vi "Get Class Types to Parent--recursive.vi"(6 "Application Ref":refnum<vi>, 7 "Class Level To Reach":refnum<class>, 8 "error in (no error)":errorcluster, 11 "Instance":refnum<class>) -> (0 "error out":errorcluster, 2 "Class Levels To Requested (FQN)":string[](array[string]), 3 "Class Levels To Requested (Types)":refnum<class>[](array[class]))   [LabVIEW 2019, in "Class Integrator.lvlib"]
uses:
  Class Integrator.lvlib
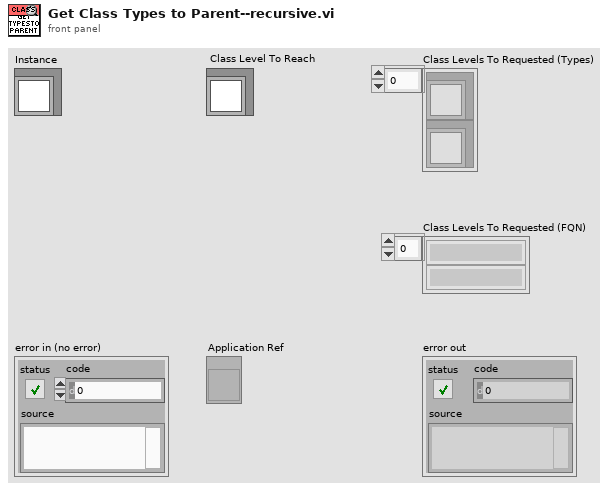
[diagram p1: front panel]
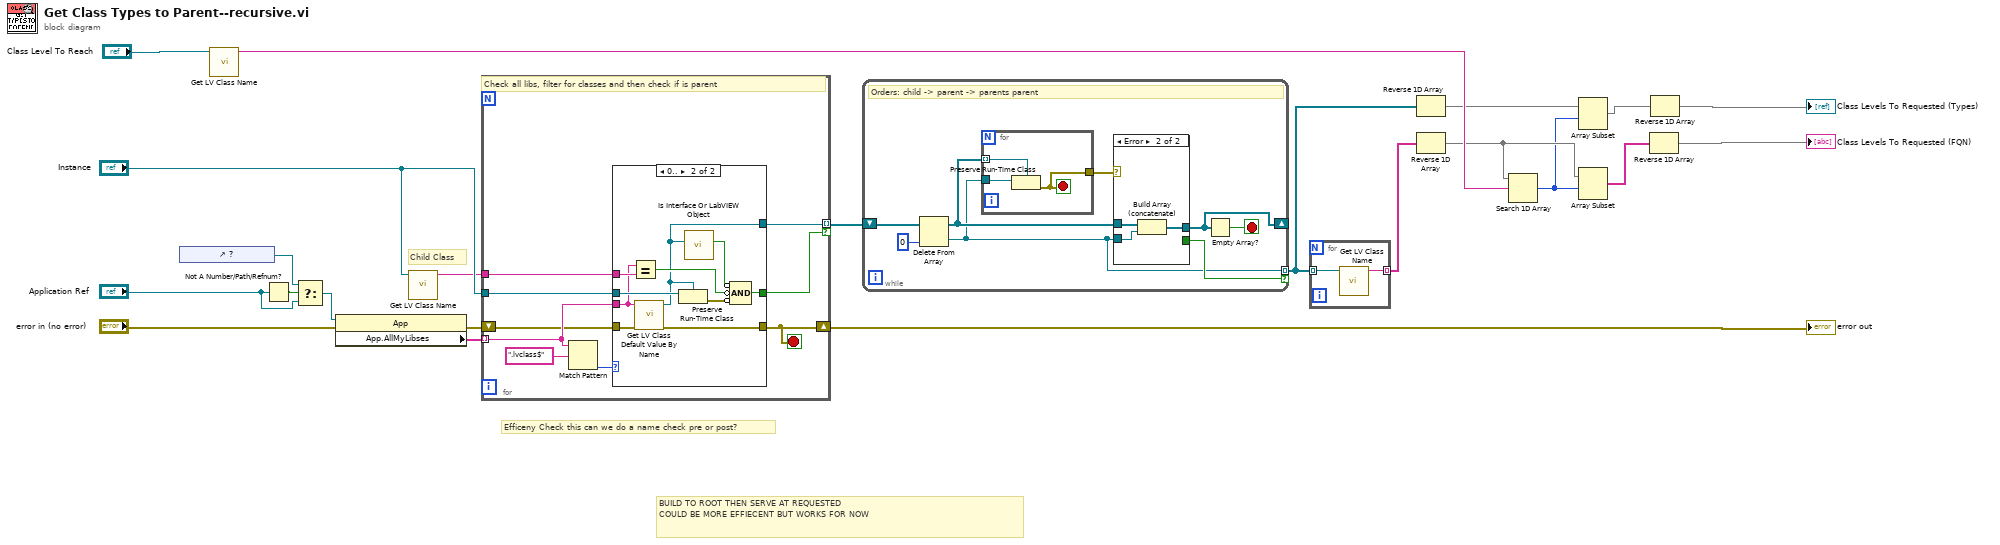
[diagram p0: block diagram]
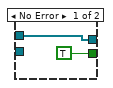
[diagram p3: hidden frame]
diagram:
  # "BUILD TO ROOT THEN SERVE AT REQUESTED\nCOULD BE MORE EFFIECENT BUT WORKS FOR NOW"
  # "Efficeny Check this can we do a name check pre or post?"
  # "Child Class"
  n1 = control-ref of="?"() -> (w14:refnum<vi>)
  n2 = call <vilib>:"Get LV Class Name.vi"("object"="Class Level To Reach") -> ("class name"=w8:string)  [unwired: 9 in, 1 out]
  n3 = Not A Number/Path/Refnum?(number/path/refnum="Application Ref") -> (NaN/Path/Refnum?=w15:bool)
  n4 = Select(t=w14, s=w15, f="Application Ref") -> (s? t:f=w9:refnum<vi>)
  n5 = property class="App"(reference=w9, error in="error in (no error)") -> (error out=w11:errorcluster, "App.AllMyLibses"=w10:string[])  [unwired: 1 out]
  n6 = call <vilib>:"Get LV Class Name.vi"("object"="Instance") -> ("class name"=w12:string)  [unwired: 9 in, 1 out]
  n7 = for {
    tunnel: w10 -> [w31] mode=indexing
    tunnel: [w26] -> w13 mode=indexing if=w25
    shift-right: [w27] -> w22
    shift-left: w11 -> [w28]
    tunnel: "Instance" -> [w24]
    tunnel: w12 -> [w23]
    stop <- w27 stop-if-true
    # "Check all libs, filter for classes and then check if is parent"
    n8 = Match Pattern(string=w31, regular expression=".lvclass$") -> (offset past match=w30:i32)  [unwired: 1 in, 3 out]
    n9 = case shown="0.." w30 {
      tunnel: [_ w33] -> w26
      tunnel: w31 -> [_ w36]
      tunnel: [_ w41] -> w25
      tunnel: [_ w40] -> w27
      tunnel: w28 -> [_ w39]
      tunnel: w24 -> [_ w38]
      tunnel: w23 -> [_ w37]
      frame Default {
      }
      frame 0.. {
        n10 = Equal?(x=w36, y=w37) -> (x = y?=w35:bool)
        n11 = call <vilib>:"Get LV Class Default Value By Name.vi"("error in (no error)"=w39, "class name"=w36) -> ("error out"=w40:errorcluster, "object"=w33:refnum<class>)  [unwired: 8 in]
        n12 = Preserve Run-Time Class(object in=w38, 2:w33) -> (error out=w34:errorcluster)  [unwired: 1 in, 1 out]
        n13 = call "Is Interface Or LabVIEW Object.vi"("LabVIEW Object"=w33) -> ("Is Interface?"=w32:bool)  [unwired: 10 in]
        n14 = Compound Arithmetic op=AND(invert w32, invert w35, invert w34) -> (w41:bool)
      }
    }
  }
  "error out" <- w22
  n15 = while {
    shift-right: [w42] -> _
    shift-left: w13 -> [w49]
    tunnel: [w43] -> w3 mode=indexing if=w44
    stop <- w46 stop-if-true
    # "Orders: child -> parent -> parents parent"
    n16 = Delete From Array(array=w49, index=0) -> (deleted portion=w43:refnum<class>, array with subset deleted=w45:refnum<class>[])  [unwired: 1 in]
    n17 = for {
      tunnel: w43 -> [w57]
      tunnel: w45 -> [w56] mode=indexing
      tunnel: [w55] -> w47
      stop <- w55 stop-if-true
      n18 = Preserve Run-Time Class(object in=w57, 2:w56) -> (error out=w55:errorcluster)  [unwired: 1 in, 1 out]
    }
    n19 = case shown="Error" w47 {
      tunnel: w45 -> [w51 w54]
      tunnel: [w51 w53] -> w42
      tunnel: [TRUE _] -> w44
      tunnel: w43 -> [_ w52]
      frame No Error {
      }
      frame Error {
        n20 = Build Array (concatenate)(w54, w52) -> (w53:refnum<class>[])
      }
    }
    n21 = Empty Array?(array=w42) -> (empty?=w46:bool)
  }
  n22 = for {
    tunnel: w3 -> [w59] mode=indexing
    tunnel: [w58] -> w7 mode=indexing
    n23 = call <vilib>:"Get LV Class Name.vi"("object"=w59) -> ("class name"=w58:string)  [unwired: 9 in, 1 out]
  }
  n24 = Reverse 1D Array(array=w3) -> (reversed array=w2:refnum<class>[])
  n25 = Reverse 1D Array(array=w7) -> (reversed array=w5:string[])
  n26 = Search 1D Array(1D array=w5, element=w8) -> (index of element=w4:i32)  [unwired: 1 in]
  n27 = Array Subset(array=w2, index=w4) -> (w1:refnum<class>[])  [unwired: 1 in]
  n28 = Array Subset(array=w5, index=w4) -> (w6:string[])  [unwired: 1 in]
  n29 = Reverse 1D Array(array=w6) -> (reversed array=→"Class Levels To Requested (FQN)":string[])
  n30 = Reverse 1D Array(array=w1) -> (reversed array=→"Class Levels To Requested (Types)":refnum<class>[])
